vi "Drop Stack Frame.vi"(8 "error in (no error)":errorcluster, 11 "gScript Interpreter in":refnum<class "gScript Interpreter.lvclass">) -> (0 "error out":errorcluster, 2 "Return Bindings":string[](array[string]), 3 "gScript Interpreter out":refnum<class "gScript Interpreter.lvclass">)   [LabVIEW 2023, in "gScript Interpreter.lvclass"]
uses:
  gScript Interpreter.lvclass
  gScript Interpreter.lvclass/gScript Interpreter.ctl
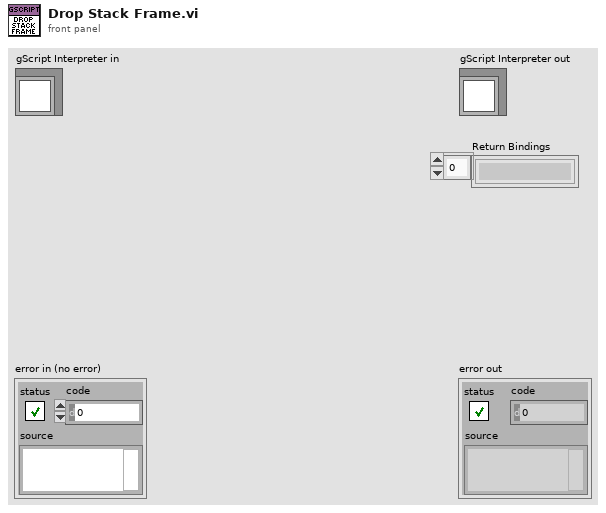
[diagram p1: front panel]
types:
  T1 = typedef "Stack Frame.ctl" = cluster{"Variable Table":T2, "Return Pointer":i32, "Return Bindings":string[]}
  T2 = typedef "Variable Table.ctl" = T3[]
  T3 = typedef "Variable.ctl" = cluster{"Variable Name":string, "Memory Cell":T4}
  T4 = typedef "Memory Cell.ctl" = cluster{"type":T5, "x":dbl, "y":dbl, "z":dbl, "w":dbl}
  T5 = typedef "Memory Cell Type Enum.ctl" = enum16{"integer", "float", "vector", "rotation"}
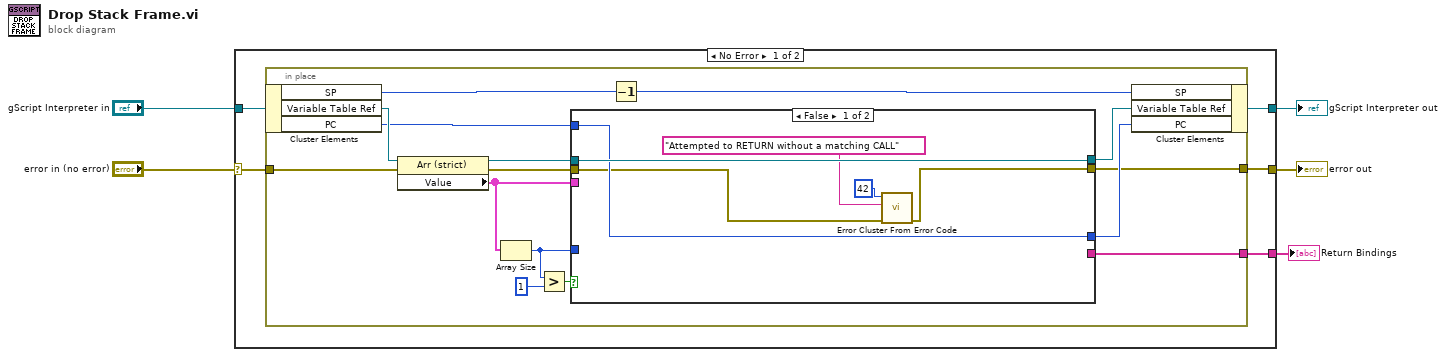
[diagram p0: block diagram]
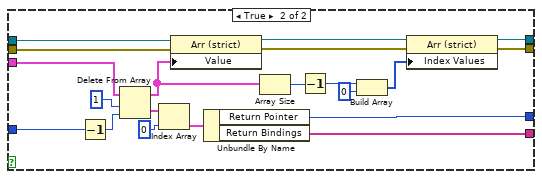
[diagram p2: hidden frame]
diagram:
  n1 = case shown="No Error" "error in (no error)" {
    selector: "error in (no error)" -> [w9 w53]
    tunnel: [w8 w53] -> w4
    tunnel: [w7 w52] -> w2
    tunnel: "gScript Interpreter in" -> [w10 w52]
    tunnel: [w6 _] -> w1
    frame No Error {
      n2 = in-place {
        in-place-border: w9 -> [w24]
        in-place-border: [w15] -> w8
        in-place-border: [w17] -> w6
        n3 = in-place-cluster #1(w10) -> ("SP"=w23:i32, "Variable Table Ref"=w25:refnum<vi>, "PC"=w11:i32)
        n4 = property class="Arr (strict)"(reference=w25, error in=w24) -> (reference out=w21:refnum<vi>, error out=w20:errorcluster, "Value"=w19:T1[])
        n5 = Array Size(array=w19) -> (size(s)=w13:i32)
        n6 = Greater?(x=w13, y=1) -> (0:w14:bool)
        n7 = case shown="False" w14 {
          tunnel: w21 -> [w31 w51]
          tunnel: w20 -> [w27 w50]
          tunnel: w19 -> [_ w48]
          tunnel: [w30 w43] -> w18
          tunnel: [_ w42] -> w17
          tunnel: [w31 w36] -> w16
          tunnel: [w29 w35] -> w15
          tunnel: w13 -> [_ w32]
          tunnel: w11 -> [w30 _]
          frame False {
            n8 = call <vilib>:"Error Cluster From Error Code.vi"("error in (no error)"=w27, "error message (\"\")"="Attempted to RETURN without a matching CALL" ("error message (\"\")"), "error code (0)"=42) -> ("error out"=w29:errorcluster)  [unwired: 6 in]
          }
          frame True {
            n9 = Decrement(x=w32) -> (x-1=w47:i32)
            n10 = Delete From Array(array=w48, length=1, index=w47) -> (deleted portion=w46:T1[], array with subset deleted=w34:T1[])
            n11 = Index Array(array=w46, index=0) -> (element=w44:T1)
            n12 = property class="Arr (strict)"(reference=w51, error in=w50, "Value"=w34) -> (reference out=w38:refnum<vi>, error out=w37:errorcluster)
            n13 = Unbundle By Name(w44) -> ("Return Pointer"=w43:i32, "Return Bindings"=w42:string[])
            n14 = Array Size(array=w34) -> (size(s)=w40:i32)
            n15 = Decrement(x=w40) -> (x-1=w39:i32)
            n16 = Build Array(w39, 0 ("element")) -> (w33:i32[])
            n17 = property class="Arr (strict)"(reference=w38, error in=w37, "Index Values"=w33) -> (reference out=w36:refnum<vi>, error out=w35:errorcluster)
          }
        }
        n18 = Decrement(x=w23) -> (x-1=w22:i32)
        n19 = in-place-cluster #1("SP"=w22, "Variable Table Ref"=w16, "PC"=w18) -> (w7:refnum<class "gScript Interpreter.lvclass">)
      }
    }
    frame Error {
    }
  }
  "error out" <- w4
  "gScript Interpreter out" <- w2
  "Return Bindings" <- w1
